vi "00 - Simplest VI(showcase).vi"() -> ()   [LabVIEW 2025]
uses:
  <vilib>/Utility/miscctls.llb/LVRectTypeDef.ctl
  Script BD FP Arrows/Arrow Direction.ctl
  5687628b-adaf-43bf-9403-46b5a02ce4fa.vi
panel:
  out "Master Bounds Rect":T1
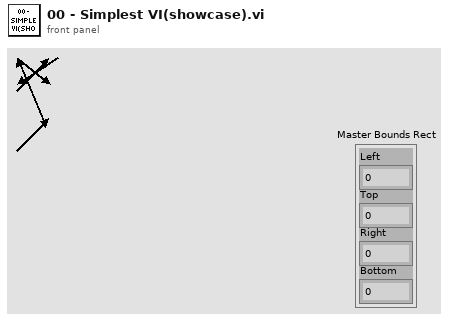
[diagram p1: front panel]
types:
  T1 = typedef "LVRectTypeDef.ctl" = cluster{"Left":i16, "Top":i16, "Right":i16, "Bottom":i16}
  T2 = typedef "Arrow Direction.ctl" = enum16{"UpRight", "UpLeft", "DownLeft", "DownRight"}
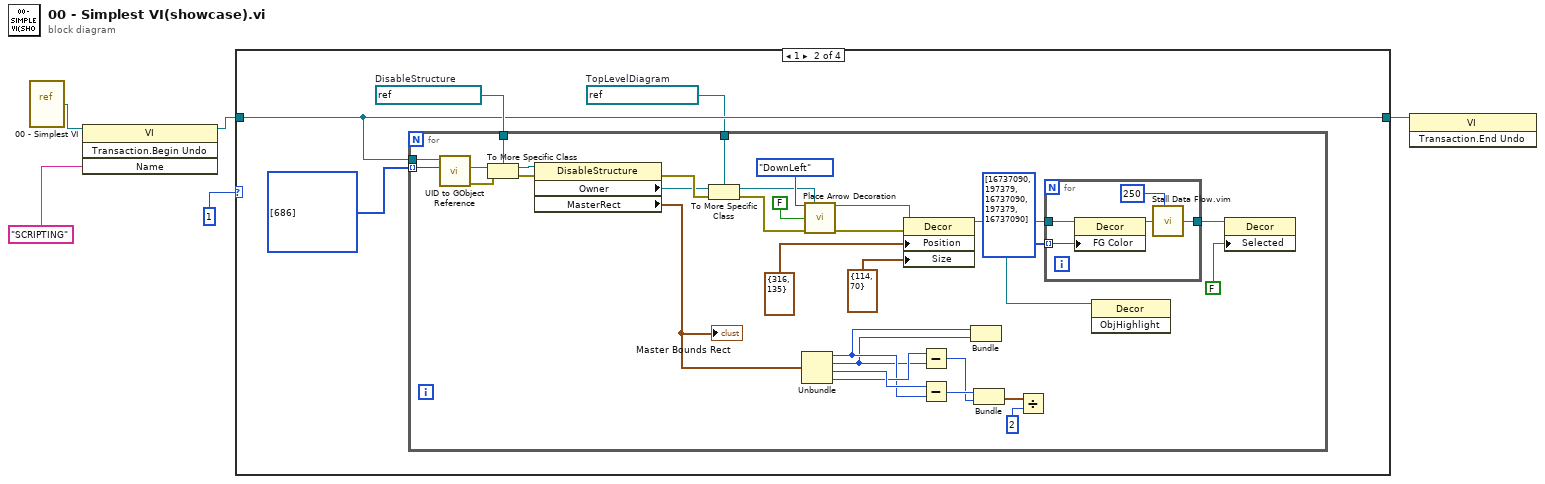
[diagram p0: block diagram]
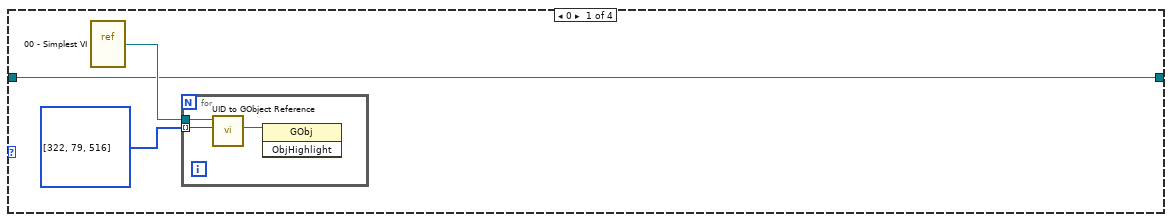
[diagram p2: hidden frame]
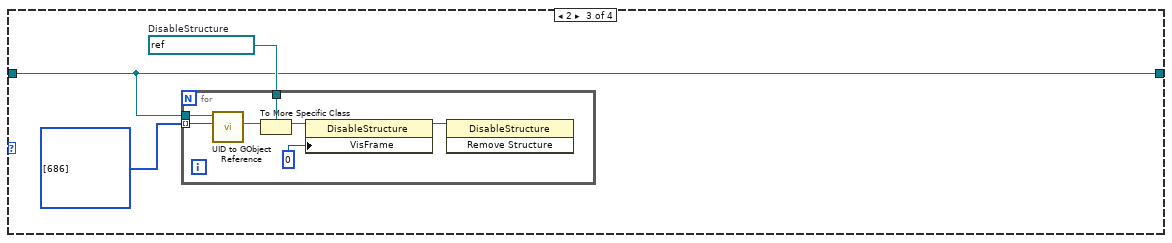
[diagram p3: hidden frame]
diagram:
  n1 = vi-ref "00 - Simplest VI.vi"() -> (w5:refnum<vi>)
  n2 = invoke class="VI" method="Transaction.Begin Undo"(reference=w5, "Name"="SCRIPTING") -> (reference out=w4:refnum<vi>)  [unwired: 2 in, 3 out]
  n3 = case shown="1" 1 ("UID") {
    tunnel: w4 -> [w6 w13 w52 w62]
    tunnel: [w6 w13 w52 w62] -> w3
    frame 0 {
      n4 = vi-ref "00 - Simplest VI.vi"() -> (w8:refnum<vi>)
      n5 = for {
        tunnel: w8 -> [w11]
        tunnel: i32[] [322, 79, 516] ("Array") -> [w10] mode=indexing
        n6 = call <vilib>:"UID to GObject Reference.vi"("UID"=w10, "Owning VI"=w11) -> ("GObject"=w9:refnum<vi>)  [unwired: 7 in, 2 out]
        n7 = invoke class="GObj" method="ObjHighlight"(reference=w9) -> ()  [unwired: 2 in, 3 out]
      }
    }
    frame 1 {
      w12 = refnum<vi> refnum  # TopLevelDiagram
      w14 = refnum<vi> refnum  # DisableStructure
      n8 = for {
        tunnel: i32[] [686] ("Array") -> [w46] mode=indexing
        tunnel: w14 -> [w44]
        tunnel: w13 -> [w43]
        tunnel: w12 -> [w37]
        n9 = call <vilib>:"UID to GObject Reference.vi"("UID"=w46, "Owning VI"=w43) -> ("error out"=w40:errorcluster, "GObject"=w45:refnum<vi>)  [unwired: 7 in, 1 out]
        n10 = To More Specific Class(target class=w44, reference=w45, error in=w40) -> (specific class reference=w42:refnum<vi>, error out=w41:errorcluster)
        n11 = property class="DisableStructure"(reference=w42, error in=w41) -> (error out=w36:errorcluster, "Owner"=w33:refnum<vi>, "MasterRect"=w24:T1)  [unwired: 1 out]
        "Master Bounds Rect" <- w24
        n12 = To More Specific Class(target class=w37, reference=w33, error in=w36) -> (specific class reference=w34:refnum<vi>, error out=w35:errorcluster)
        n13 = Unbundle(w24) -> ("Left"=w26:i16, "Top"=w25:i16, "Right"=w32:i16, "Bottom"=w31:i16)
        n14 = call "Place Arrow Decoration.vi"("Arrow Direction"=Arrow_Direction."DownLeft", "Diagram"=w34, "FP? (T)"=FALSE, "error in"=w35) -> ("Decor Refnum"=w22:refnum<vi>, "error out"=w23:errorcluster)  [unwired: 10 in]
        n15 = property class="Decor"(reference=w22, error in=w23, "Position"=cluster{"Left":i32, "Top":i32} {"Left"=316, "Top"=135}, "Size"=cluster{"Width":u32, "Height":u32} {"Width"=114, "Height"=70}) -> (reference out=w18:refnum<vi>)  [unwired: 1 out]
        n16 = Subtract(x=w31, y=w25) -> (x-y=w29:i16)
        n17 = Subtract(x=w32, y=w26) -> (x-y=w30:i16)
        n18 = Bundle("Left"=w26, "Top"=w25) -> ()  [unwired: 1 in, 1 out]
        n19 = Bundle(w30, w29) -> (w28:cluster{i16, i16})  [unwired: 1 in]
        n20 = Divide(x=w28, y=2 ("UID")) -> ()  [unwired: 1 out]
        n21 = for {
          tunnel: w18 -> [w51]
          tunnel: u32[] [16737090, 197379, 16737090, 197379, 16737090] -> [w50] mode=indexing
          tunnel: [w48] -> w17
          n22 = property class="Decor"(reference=w51, "FG Color"=w50) -> (reference out=w49:refnum<vi>)  [unwired: 1 in, 1 out]
          n23 = call "Stall Data Flow.vim"("value in"=w49, "milliseconds to wait"=u32 250) -> ("value out"=w48:refnum<vi>)  [unwired: 1 out]
        }
        n24 = invoke class="Decor" method="ObjHighlight"(reference=w18) -> ()  [unwired: 2 in, 3 out]
        n25 = property class="Decor"(reference=w17, "Selected"=FALSE) -> ()  [unwired: 1 in, 2 out]
      }
    }
    frame 2 {
      w53 = refnum<vi> refnum  # DisableStructure
      n26 = for {
        tunnel: i32[] [686] ("Array") -> [w61] mode=indexing
        tunnel: w53 -> [w58]
        tunnel: w52 -> [w57]
        n27 = call <vilib>:"UID to GObject Reference.vi"("UID"=w61, "Owning VI"=w57) -> ("GObject"=w60:refnum<vi>)  [unwired: 7 in, 2 out]
        n28 = To More Specific Class(target class=w58, reference=w60) -> (specific class reference=w59:refnum<vi>)  [unwired: 1 in, 1 out]
        n29 = property class="DisableStructure"(reference=w59, "VisFrame"=u32 0 ("Visible Frame")) -> (reference out=w56:refnum<vi>)  [unwired: 1 in, 1 out]
        n30 = invoke class="DisableStructure" method="Remove Structure"(reference=w56) -> ()  [unwired: 2 in, 3 out]
      }
    }
    frame Default {
    }
  }
  n31 = invoke class="VI" method="Transaction.End Undo"(reference=w3) -> ()  [unwired: 2 in, 3 out]
